vi "DisplacementCalc_171213.vi"(7 "TotalDistanceTraveledInput":dbl, 9 "i":i32, 10 "Y":dbl, 11 "X":dbl) -> (1 "Speed":dbl, 2 "TotalDistanceTraveledOutput":dbl)   [LabVIEW 2016]
panel:
  out "Y old":dbl
  out "X old":dbl
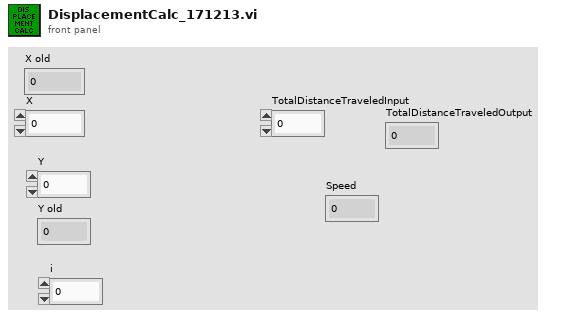
[diagram p1: front panel]
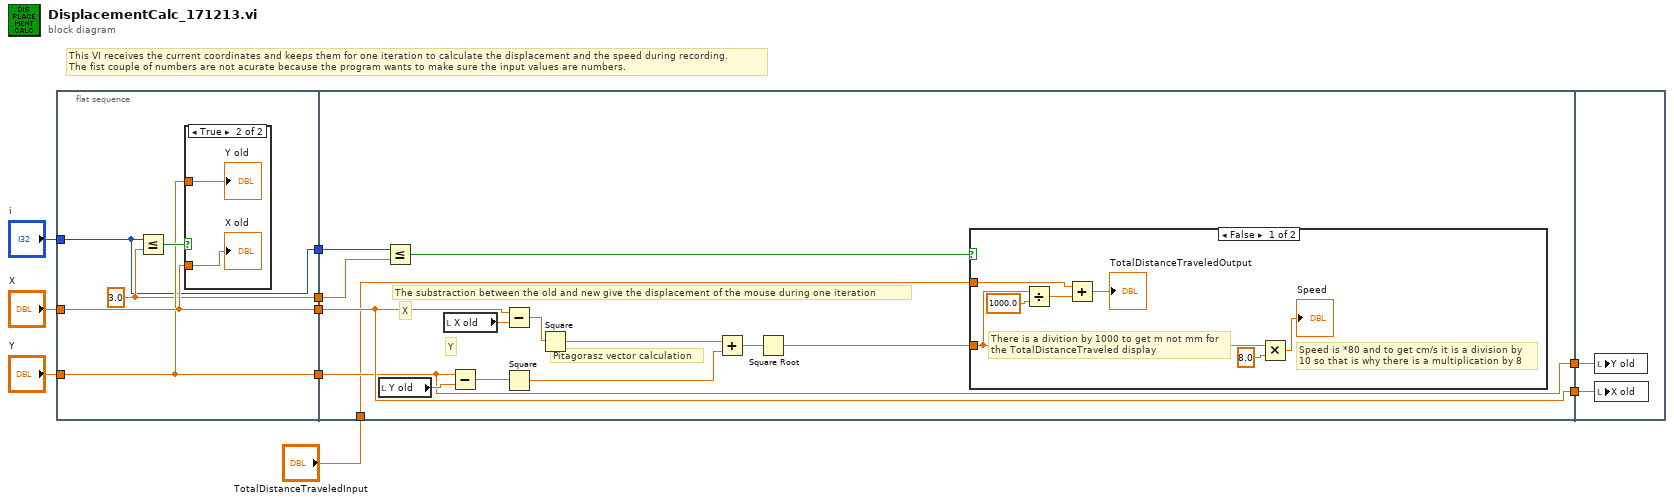
[diagram p0: block diagram]
diagram:
  # "This VI receives the current coordinates and keeps them for one iteration to calculate the displacement and the speed during recording.\nThe fist couple of numbers are not acurate because the program wants to make sure the input values are numbers."
  n1 = flat-sequence {
    tunnel: "Y" -> [w13]
    tunnel: "X" -> [w14]
    tunnel: [w14] -> w6
    tunnel: [w13] -> w5
    tunnel: "i" -> [w11]
    tunnel: [w12] -> w2
    tunnel: [w11] -> w1
    tunnel: [w23] -> w10
    tunnel: [w24] -> w9
    tunnel: w6 -> [w24]
    tunnel: w5 -> [w23]
    tunnel: "TotalDistanceTraveledInput" -> [w22]
    tunnel: w2 -> [w19]
    tunnel: w1 -> [w18]
    tunnel: w10 -> [w39]
    tunnel: w9 -> [w40]
    frame #0 {
      w12 = 3.0 ("y")
      n2 = Less Or Equal?(x=w11, y=w12) -> (x <= y?=w15:bool)
      n3 = case shown="True" w15 {
        tunnel: w14 -> [_ w17]
        tunnel: w13 -> [_ w16]
        frame False {
        }
        frame True {
          "X old" <- w17
          "Y old" <- w16
        }
      }
    }
    frame #1 {
      # "The substraction between the old and new give the displacement of the mouse during one iteration"
      # "Pitagorasz vector calculation"
      # "X"
      # "Y"
      n4 = local read "Y old"() -> (w31:dbl)
      n5 = Less Or Equal?(x=w18, y=w19) -> (x <= y?=w20:bool)
      n6 = local read "X old"() -> (w30:dbl)
      n7 = Subtract(x=w23, y=w31) -> (x-y=w25:dbl)
      n8 = Subtract(x=w24, y=w30) -> (x-y=w26:dbl)
      n9 = Square(x=w25) -> (x^2=w28:dbl)
      n10 = Square(x=w26) -> (x^2=w27:dbl)
      n11 = Add(x=w27, y=w28) -> (x+y=w29:dbl)
      n12 = Square Root(x=w29) -> (sqrt(x)=w21:dbl)
      n13 = case shown="False" w20 {
        tunnel: w22 -> [w36 _]
        tunnel: w21 -> [w32 _]
        frame False {
          # "There is a divition by 1000 to get m not mm for\nthe TotalDistanceTraveled display"
          # "Speed is *80 and to get cm/s it is a division by \n10 so that is why there is a multiplication by 8"
          n14 = Divide(x=w32, y=1000.0) -> (x/y=w37:dbl)
          n15 = Add(x=w36, y=w37) -> (x+y=→"TotalDistanceTraveledOutput":dbl)
          n16 = Multiply(x=w32, y=8.0) -> (x*y=→"Speed":dbl)
        }
        frame True {
        }
      }
    }
    frame #2 {
      n17 = local write "Y old"(w39) -> ()
      n18 = local write "X old"(w40) -> ()
    }
  }
